vi "Goal Vision Calculations V3.vi"(10 "Target Height (in)":dbl) -> (0 "Y Angle":dbl, 1 "X Angle":dbl, 3 "Distance (in)":dbl)   [LabVIEW 2016]
uses:
  <vilib>/Rock Robotics/Network Tables/NT Read Number.vi
panel:
  in  "X axis field of view (deg)":dbl=61.0
  in  "Image width(px)":dbl=320.0
  in  "Y axis field of view (deg)":dbl=34.3
  in  "Image height (px)":dbl=240.0
  in  "Camera Angle (deg)":dbl=11.0
  in  "Camera Height (in)":dbl=21.0
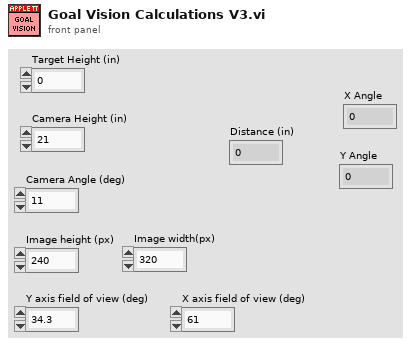
[diagram p1: front panel]
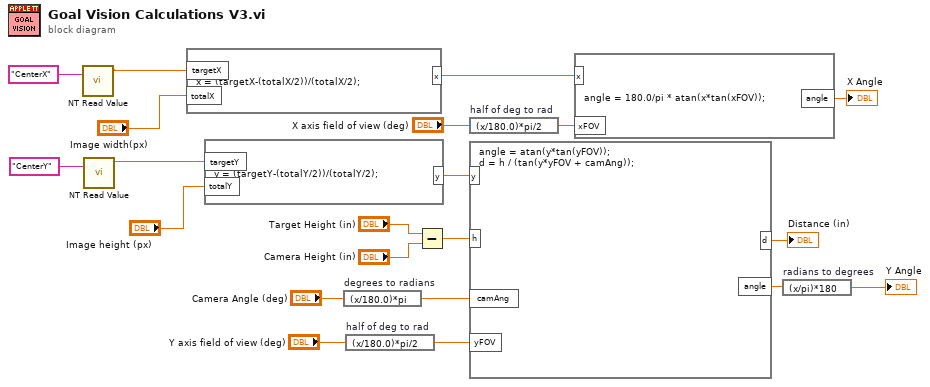
[diagram p0: block diagram]
diagram:
  n1 = call-poly <vilib>:"NT Read Value.vi"("Name"="CenterX") -> ("Numeric"=w7:dbl)  [unwired: 9 in, 1 out]
  n2 = call-poly <vilib>:"NT Read Value.vi"("Name"="CenterY") -> ("Numeric"=w9:dbl)  [unwired: 9 in, 1 out]
  n3 = formula code="x = (targetX-(totalX/2))/(totalX/2);"("targetX"=w7, "totalX"="Image width(px)") -> ("x"=w4:dbl)
  n4 = formula code="y = (targetY-(totalY/2))/(totalY/2);"("targetY"=w9, "totalY"="Image height (px)") -> ("y"=w11:dbl)
  n5 = expression code="(x/180.0)*pi" "degrees to radians"("Camera Angle (deg)") -> (w13:dbl)
  n6 = expression code="(x/180.0)*pi/2" "half of deg to rad"("Y axis field of view (deg)") -> (w14:dbl)
  n7 = Subtract(x="Target Height (in)", y="Camera Height (in)") -> (x-y=w12:dbl)
  n8 = expression code="(x/180.0)*pi/2" "half of deg to rad"("X axis field of view (deg)") -> (w5:dbl)
  n9 = formula code="angle = atan(y*tan(yFOV));\nd = h / (tan(y*yFOV + camAng));"("y"=w11, "h"=w12, "camAng"=w13, "yFOV"=w14) -> ("d"=→"Distance (in)":dbl, "angle"=w2:dbl)
  n10 = formula code="angle = 180.0/pi * atan(x*tan(xFOV));"("xFOV"=w5, "x"=w4) -> ("angle"=→"X Angle":dbl)
  n11 = expression code="(x/pi)*180" "radians to degrees"(w2) -> (→"Y Angle":dbl)
